vi "CheckState.vi"(8 "Error In":errorcluster, 10 "With sound?":bool, 11 "BattleDroid in":refnum<class "BattleDroid.lvclass">) -> (0 "Error Out":errorcluster, 3 "BattleDroid out":refnum<class "BattleDroid.lvclass">)   [LabVIEW 2021, in "BattleDroid.lvclass"]
uses:
  BattleDroid.lvclass
  Droid/Droid.lvclass
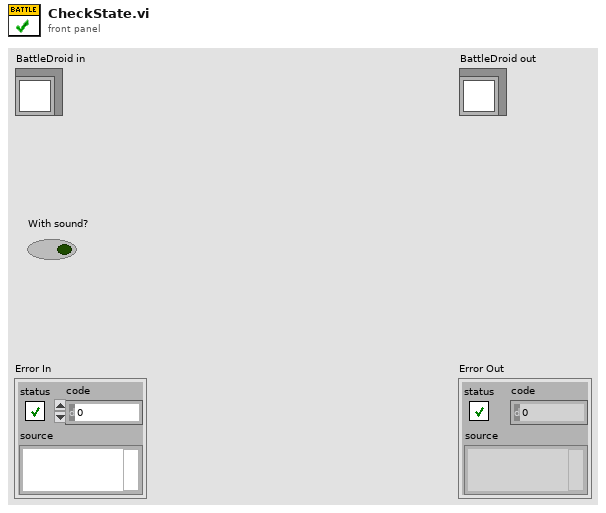
[diagram p1: front panel]
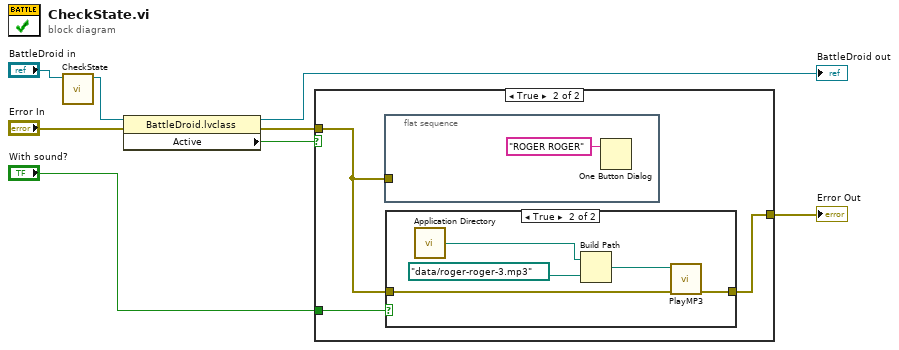
[diagram p0: block diagram]
diagram:
  n1 = call-parent "CheckState.vi"("Droid in"="BattleDroid in") -> ("Droid out"=w1:refnum<class "BattleDroid.lvclass">)  [unwired: 9 in, 1 out]
  n2 = property class="BattleDroid.lvclass"(reference=w1, error in="Error In") -> (reference out=→"BattleDroid out":refnum<class "BattleDroid.lvclass">, error out=w7:errorcluster, "Active"=w8:bool)
  n3 = case shown="True" w8 {
    tunnel: [w9 w12] -> w3
    tunnel: "With sound?" -> [_ w10]
    tunnel: w7 -> [w9 w11]
    frame False {
    }
    frame True {
      n4 = flat-sequence {
        tunnel: w11 -> [_]
        frame #0 {
          n5 = One Button Dialog(message="ROGER ROGER") -> ()  [unwired: 1 in, 1 out]
        }
      }
      n6 = case shown="True" w10 {
        tunnel: w11 -> [w14 w16]
        tunnel: [w14 w15] -> w12
        frame False {
        }
        frame True {
          n7 = call <vilib>:"Application Directory.vi"() -> ("Application Directory"=w17:path)
          n8 = Build Path(base path=w17, name or relative path=path "data/roger-roger-3.mp3") -> (appended path=w19:path)
          n9 = call "PlayMP3.vi"("Error In"=w16, "Path"=w19) -> ("Error out"=w15:errorcluster)  [unwired: 9 in]
        }
      }
    }
  }
  "Error Out" <- w3
